vi "iRobot UART Bytes at Port.vi"(8 "error in":errorcluster, 11 "UART port in":T1) -> (0 "error out":errorcluster, 1 "bytes at port":u32, 3 "UART port out":T1)   [LabVIEW 2010]
doc: "Return the number of bytes in the UART receive buffer."
uses:
  UART Port Type.ctl
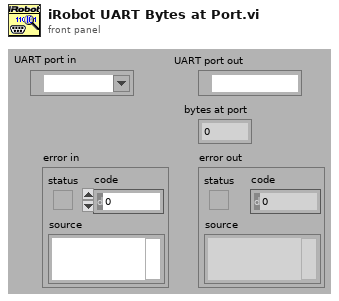
[diagram p1: front panel]
types:
  T1 = typedef "UART Port Type.ctl" = refnum<visa-resource-name>
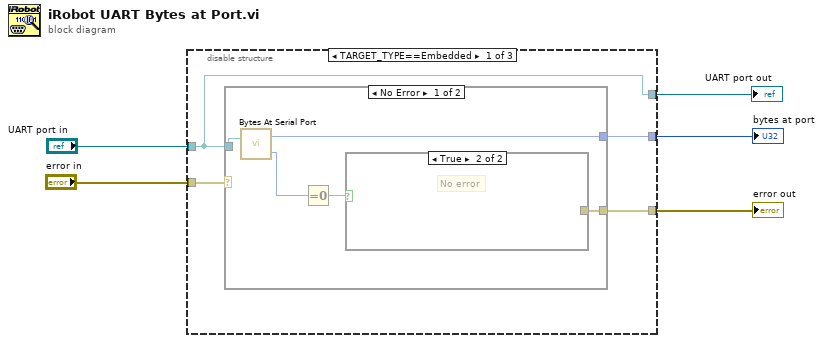
[diagram p0: block diagram]
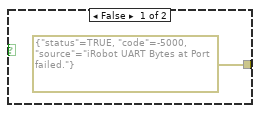
[diagram p2: hidden frame]
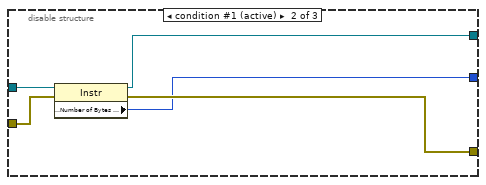
[diagram p4: hidden frame]
diagram:
  n1 = disable-structure shown="TARGET_TYPE==Embedded" {
    disable-tunnel: "UART port in" -> [w6 w21 _]
    disable-tunnel: [w9 w18 _] -> w4
    disable-tunnel: "error in" -> [w8 w20 _]
    disable-tunnel: [w7 w17 _] -> w2
    disable-tunnel: [w6 w19 _] -> w1
    frame condition #0 {
      n2 = case shown="No Error" w8 {
        selector: w8 -> [_ w16]
        tunnel: w6 -> [w14 _]
        tunnel: [w11 w16] -> w9
        tunnel: [w10 _] -> w7
        frame No Error {
          n3 = call <vilib>:"Bytes At Serial Port.vi"("port number"=w14) -> ("byte count"=w10:u32, "error code"=w13:i32)
          n4 = Equal To 0?(x=w13) -> (x = 0?=w12:bool)
          n5 = case shown="True" w12 {
            tunnel: [errorcluster {"status"=TRUE, "code"=-5000, "source"="iRobot UART Bytes at Port failed."} ("error out") _] -> w11
            frame False {
            }
            frame True {
              # "No error"
            }
          }
        }
        frame Error {
        }
      }
    }
    frame condition #1 (active) {
      n6 = property class="Instr"(reference=w21, error in=w20) -> (reference out=w19:T1, error out=w18:errorcluster, "Serial Settings:Number of Bytes at Serial Port"=w17:u32)
    }
    frame condition #2 {
      # "To be deployed..."
    }
  }
  "UART port out" <- w1
  "error out" <- w4
  "bytes at port" <- w2
